vi "Test Passing Fail If Equal Test.vi"(8 "error in (no error)":errorcluster, 11 "LUnit Test Case V2 Test Double In":refnum<class "LUnit Test Case V2 Test Double.lvclass">) -> (0 "error out":errorcluster, 3 "LUnit Test Case V2 Test Double Out":refnum<class "LUnit Test Case V2 Test Double.lvclass">)   [LabVIEW 2020, in "LUnit Test Case V2 Test Double.lvclass"]
uses:
  LUnit Test Case V2 Test Double.lvclass
  C:/Git/astemes-lunit/source/Rewrite Project/LUnit Test Case/LUnit Test Case V2.lvclass
  LUnit Test Case/LUnit Test Case V2.lvclass/LUnit Test Case V2.ctl
  e95be6d6-2f47-4a99-babb-488ecb90647c.vi
  LUnit Test Case/Private/Append Fail Result.vi
  LUnit Test Case/Private/Append Pass Result.vi
  LUnit Test Case/Private/Compare Variants.vi
  LUnit Test Case/Private/Describe Comparison.vi
  LUnit Test Case/Private/Variant to string.vi
  <vilib>/Utility/Data Type/Get Type Information.vi
  <vilib>/Utility/LVClass/Get LV Class Name.vi
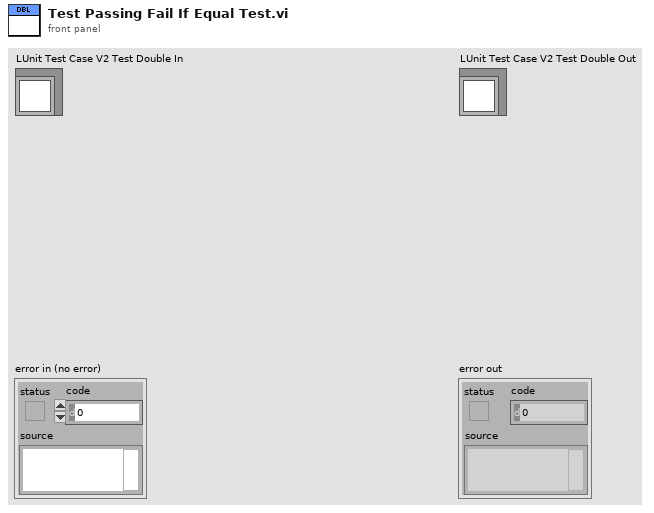
[diagram p1: front panel]
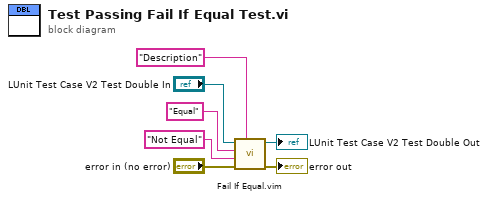
[diagram p0: block diagram]
diagram:
  n1 = call "Fail If Equal.vim"("Description"="Description", "error in (no error)"="error in (no error)", "Actual"="Not Equal", "Expected"="Equal", "LUnit Test Case In"="LUnit Test Case V2 Test Double In") -> ("error out"=→"error out":errorcluster, "LUnit Test Case Out"=→"LUnit Test Case V2 Test Double Out":refnum<class "LUnit Test Case V2 Test Double.lvclass">)  [unwired: 5 in]
